vi "CSMSVMgr Read INI String.vi"(6 "Force Default Session?(F)":bool, 8 "error in (no error)":errorcluster, 9 "Default":string, 10 "Variable Name":string, 11 "CSM-Static-Variable-Manager in":refnum<class "CSM-Static-Variable-Manager.lvclass">) -> (0 "error out":errorcluster, 1 "Content":string, 2 "Key Replaced?":bool, 3 "CSM-Static-Variable-Manager out":refnum<class "CSM-Static-Variable-Manager.lvclass">)   [LabVIEW 2017, in "INI-Static-Variable-Support.lvlib" / "CSM-Static-Variable-Manager.lvclass"]
uses:
  CSM-Static-Variable-Manager.lvclass
  CSM-Static-Variable-Manager.lvclass/CSM-Static-Variable-Manager.ctl
  INI-Static-Variable-Support.lvlib
  LabVIEW-Config/LabVIEW-Config.lvlib
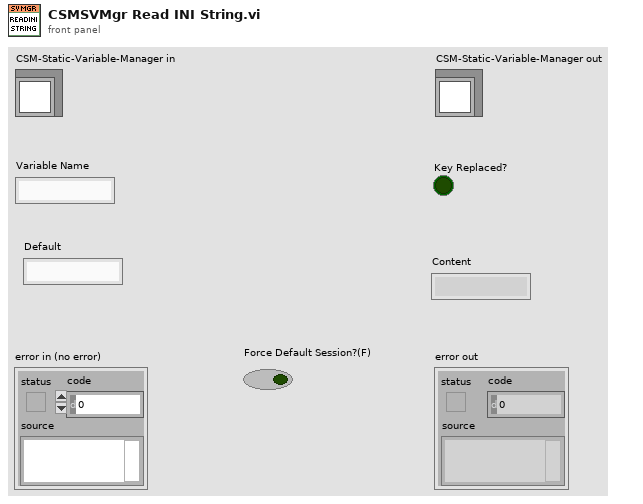
[diagram p1: front panel]
types:
  T1 = typedef "LabVIEW-Config.lvlib/Config.ctl" = cluster{"Path":path, "Lines":string[], "Tokens":T2[], "Modified?":bool}
  T2 = typedef "LabVIEW-Config.lvlib/LineToken.ctl" = enum8{"comment", "section", "key", "more"}
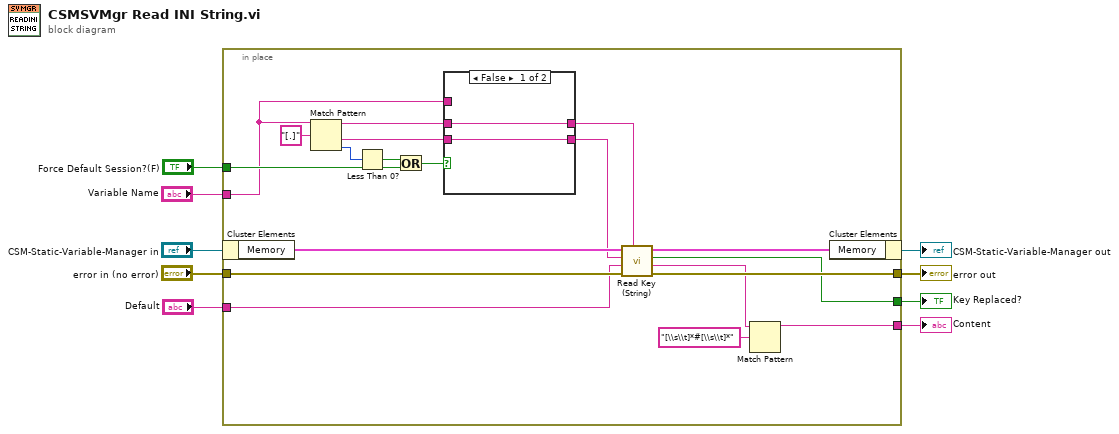
[diagram p0: block diagram]
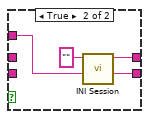
[diagram p2: hidden frame]
diagram:
  n1 = in-place {
    in-place-border: "error in (no error)" -> [w26]
    in-place-border: [w25] -> w6
    in-place-border: [w24] -> w5
    in-place-border: "Variable Name" -> [w16]
    in-place-border: "Force Default Session?(F)" -> [w20]
    in-place-border: [w10] -> w2
    in-place-border: "Default" -> [w13]
    n2 = in-place-cluster #1("CSM-Static-Variable-Manager in") -> ("Memory"=w28:T1)
    n3 = Match Pattern(string=w16, regular expression="[.]") -> (before substring=w17:string, after substring=w15:string, offset past match=w22:i32)  [unwired: 1 in, 1 out]
    n4 = Less Than 0?(x=w22) -> (x < 0?=w21:bool)
    n5 = Or(x=w21, y=w20) -> (x .or. y?=w19:bool)
    n6 = case shown="False" w19 {
      tunnel: [w30 w33] -> w18
      tunnel: w17 -> [w30 _]
      tunnel: w16 -> [_ w32]
      tunnel: w15 -> [w29 _]
      tunnel: [w29 w32] -> w14
      frame False {
      }
      frame True {
        n7 = call "INI Session.vi"("Section Name(\"\" as Default)"="" ("Section Name(\"\" as Default)")) -> ("App.Name"=w33:string)  [unwired: 10 in]
      }
    }
    n8 = call "Read Key (String).vi"("Section Name"=w18, "error in (no error)"=w26, "Default"=w13, "Key Name"=w14, "Config in"=w28) -> ("error out"=w25:errorcluster, "Value"=w12:string, "Key Found?"=w24:bool, "Config out"=w27:T1)  [unwired: 3 in]
    n9 = Match Pattern(string=w12, regular expression="[\\s\\t]*#[\\s\\t]*") -> (before substring=w10:string)  [unwired: 1 in, 3 out]
    n10 = in-place-cluster #1("Memory"=w27) -> (→"CSM-Static-Variable-Manager out":refnum<class "CSM-Static-Variable-Manager.lvclass">)
  }
  "error out" <- w6
  "Key Replaced?" <- w5
  "Content" <- w2
